vi "checkFinishZigZagPlay.vi"(8 "error in (no error)":errorcluster, 10 "Game":refnum<class "Game.lvclass">, 11 "ZigZagPlay in":refnum<class "ZigZagPlay.lvclass">) -> (0 "error out":errorcluster, 2 "Boolean":bool, 3 "ZigZagPlay out":refnum<class "ZigZagPlay.lvclass">)   [LabVIEW 2023, in "ZigZagPlay.lvclass"]
uses:
  ZigZagPlay.lvclass
  Game_class/Game.lvclass
  Game_class/Game.lvclass/Game.ctl
  Game_class/Read TestMode.vi
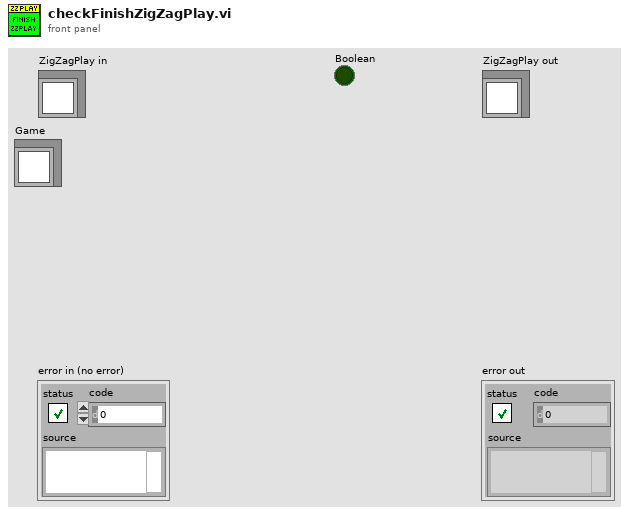
[diagram p1: front panel]
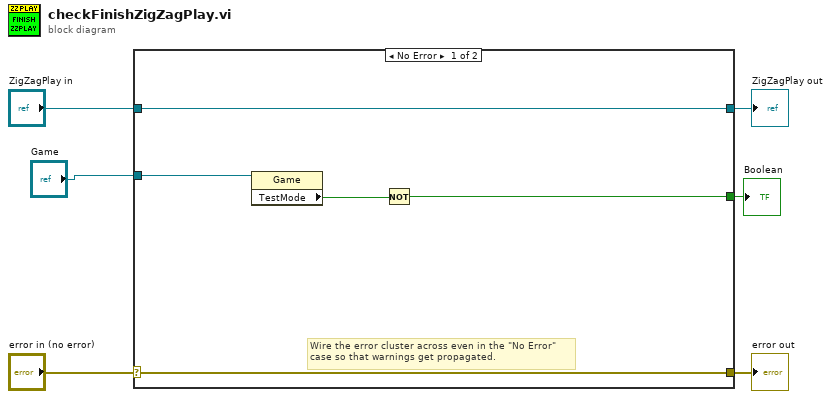
[diagram p0: block diagram]
diagram:
  n1 = case shown="No Error" "error in (no error)" {
    selector: "error in (no error)" -> [w10 w13]
    tunnel: [w10 w13] -> w5
    tunnel: [w11 w12] -> w3
    tunnel: "ZigZagPlay in" -> [w11 w12]
    tunnel: "Game" -> [w9 _]
    tunnel: [w7 _] -> w1
    frame No Error {
      # "Wire the error cluster across even in the \"No Error\"\ncase so that warnings get propagated."
      n2 = property class="Game"(reference=w9) -> ("TestMode"=w8:bool)  [unwired: 1 in, 2 out]
      n3 = Not(x=w8) -> (.not. x?=w7:bool)
    }
    frame Error {
    }
  }
  "error out" <- w5
  "ZigZagPlay out" <- w3
  "Boolean" <- w1
